vi "Read Frame.vi"(8 "error in (no error)":errorcluster, 11 "TroSpec in":refnum<class "PL ISTEQ TroSpec.lvclass">) -> (0 "error out":errorcluster, 1 "lost frames":u16, 2 "frame":u32[](array[numeric]), 3 "TroSpec out":refnum<class "PL ISTEQ TroSpec.lvclass">)   [LabVIEW 2015, in "PL ISTEQ TroSpec.lvclass"]
doc: "Reads single frame. Should be called after the Start Acquisition.vi."
uses:
  PL ISTEQ TroSpec.lvclass
  PL ISTEQ TroSpec.lvclass/PL ISTEQ TroSpec.ctl
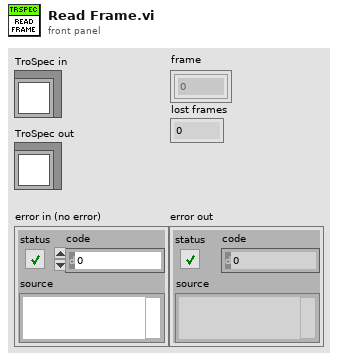
[diagram p1: front panel]
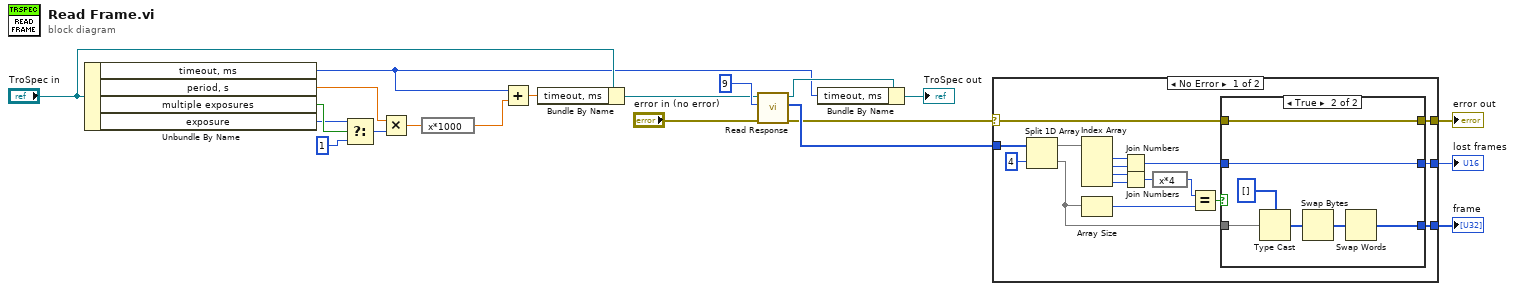
[diagram p0: block diagram]
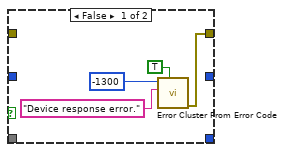
[diagram p2: hidden frame]
diagram:
  n1 = Unbundle By Name("TroSpec in") -> ("timeout, ms"=w9:u32, "period, s"=w4:dbl, "multiple exposures"=w8:bool, "exposure"=w7:u32)
  n2 = Select(t=w7, s=w8, f=u32 1) -> (s? t:f=w5:u32)
  n3 = Multiply(x=w4, y=w5) -> (x*y=w3:dbl)
  n4 = expression code="x*1000"(w3) -> (w2:dbl)
  n5 = Add(x=w9, y=w2) -> (x+y=w1:dbl)
  n6 = Bundle By Name(cluster="TroSpec in", "timeout, ms"=w1) -> (w12:refnum<class "PL ISTEQ TroSpec.lvclass">)
  n7 = call "Read Response.vi"("error in (no error)"="error in (no error)", "command"=u8 9, "TroSpec in"=w12) -> ("error out"=w16:errorcluster, "response payload"=w18:u8[], "TroSpec out"=w10:refnum<class "PL ISTEQ TroSpec.lvclass">)  [unwired: 6 in]
  n8 = Bundle By Name(cluster=w10, "timeout, ms"=w9) -> (→"TroSpec out":refnum<class "PL ISTEQ TroSpec.lvclass">)
  n9 = case shown="No Error" w16 {
    selector: w16 -> [w24 w49]
    tunnel: w18 -> [w37 _]
    tunnel: [w35 _] -> w17
    tunnel: [w25 w49] -> w15
    tunnel: [w26 _] -> w14
    frame No Error {
      n10 = Split 1D Array(array=w37, index=4) -> (first subarray=w34:u8[], second subarray=w29:u8[])
      n11 = Index Array(array=w34) -> (element #1=w33:u8, element #2=w32:u8, element #3=w30:u8, element #4=w31:u8)  [unwired: 4 in]
      n12 = Array Size(array=w29) -> (size(s)=w23:i32)
      n13 = Join Numbers(hi=w33, lo=w32) -> ((hi.lo)=w28:u16)
      n14 = Join Numbers(hi=w30, lo=w31) -> ((hi.lo)=w22:u16)
      n15 = expression code="x*4"(w22) -> (w21:u16)
      n16 = Equal?(x=w21, y=w23) -> (x = y?=w27:bool)
      n17 = case shown="True" w27 {
        tunnel: [_ w42] -> w35
        tunnel: w29 -> [_ w46]
        tunnel: w28 -> [_ w45]
        tunnel: [_ w45] -> w26
        tunnel: [w38 w44] -> w25
        tunnel: w24 -> [_ w44]
        frame False {
          n18 = call <vilib>:"Error Cluster From Error Code.vi"("show call chain? (False)"=TRUE, "error message (\"\")"="Device response error." ("format string"), "error code (0)"=-1300) -> ("error out"=w38:errorcluster)  [unwired: 6 in]
        }
        frame True {
          n19 = Type Cast(type=u32[] [] ("frame"), x=w46) -> (*(type *) &x=w47:u32[])
          n20 = Swap Bytes(anything=w47) -> (byte swapped=w43:u32[])
          n21 = Swap Words(1:w43) -> (0:w42:u32[])
        }
      }
    }
    frame Error {
    }
  }
  "error out" <- w15
  "frame" <- w17
  "lost frames" <- w14
